vi "Thor_CloseDevice.vi"(7 "shutDown Device?":bool=TRUE, 8 "error in (no error)":errorcluster, 10 "Device In":T1, 11 "KCubeServoControl In":T2) -> (0 "error out":errorcluster, 2 "Device Out":T1, 5 "CloseDevice":bool)   [LabVIEW 2020]
uses:
  Thor_DeviceRef.ctl
  E:/Norway Project/All Hardware/New Microscope/LabVIEW/ThorLabs/ThorLabs.MotionControl.KCube.DCServoCLI.dll
  ThorLabs.MotionControl.KCube.DCServoCLI.dll
  Thor_KCubeServoDCRef.ctl
  E:/Norway Project/All Hardware/New Microscope/LabVIEW/ThorLabs/Thorlabs.MotionControl.Controls.dll
  Thorlabs.MotionControl.Controls.dll
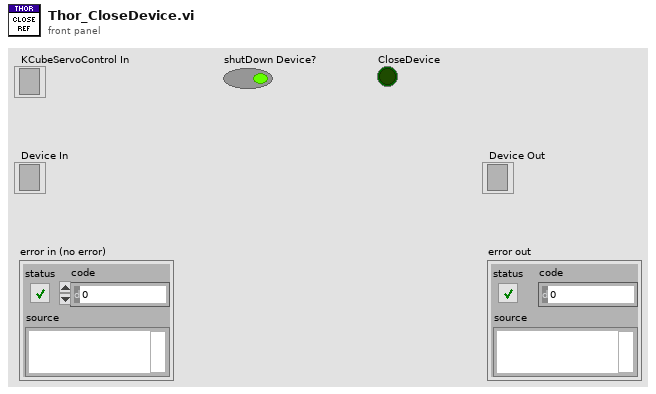
[diagram p1: front panel]
types:
  T1 = typedef "Thor_DeviceRef.ctl" = refnum<k24>
  T2 = typedef "Thor_KCubeServoDCRef.ctl" = refnum<k24>
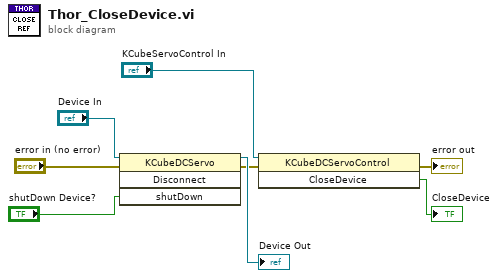
[diagram p0: block diagram]
diagram:
  n1 = invoke class="KCubeDCServo" method="Disconnect"(reference="Device In", error in="error in (no error)", "shutDown"="shutDown Device?") -> (reference out=→"Device Out":T1, error out=w1:errorcluster)  [unwired: 1 in, 2 out]
  n2 = invoke class="KCubeDCServoControl" method="CloseDevice"(reference="KCubeServoControl In", error in=w1) -> (error out=→"error out":errorcluster, "CloseDevice"=→"CloseDevice":bool)  [unwired: 1 in, 1 out]
